vi "Source_File and folder names.vi"() -> (0 "Fixed strings":T1)   [LabVIEW 2020]
uses:
  Typedefs/Fixed strings.ctl
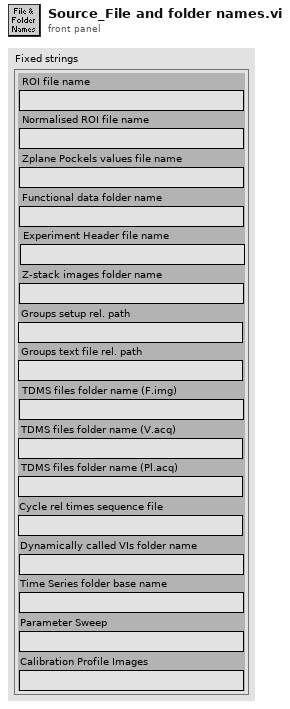
[diagram p1: front panel]
types:
  T1 = typedef "Fixed strings.ctl" = cluster{"ROI file name":string, "Normalised ROI file name":string, "Zplane Pockels values file name":string, "Functional data folder name":string, "Experiment Header file name":string, "Z-stack images folder name":string, "Groups setup rel. path":string, "Groups text file rel. path":string, "TDMS files folder name (F.img)":string, "TDMS files folder name (V.acq)":string, "TDMS files folder name (Pl.acq)":string, "Cycle rel times sequence file":string, "Dynamically called VIs folder name":string, "Time Series folder base name":string, "Parameter Sweep":string, "Calibration Profile Images":string}
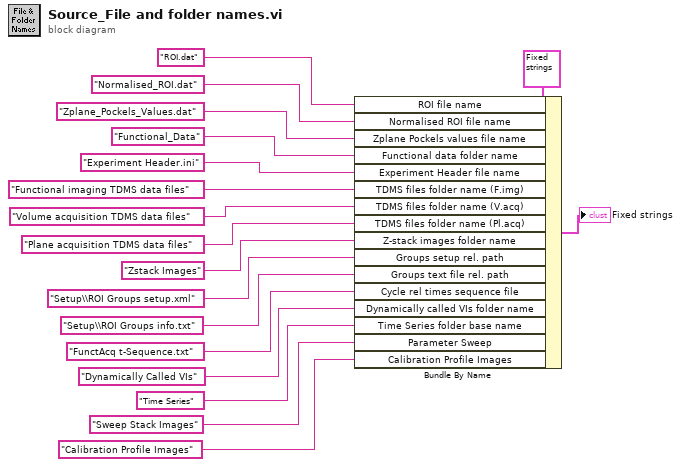
[diagram p0: block diagram]
diagram:
  n1 = Bundle By Name(cluster=T1 {"ROI file name"="", "Normalised ROI file name"="", "Zplane Pockels values file name"="", "Functional data folder name"="", "Experiment Header file name"="", "Z-stack images folder name"="", "Groups setup rel. path"="", "Groups text file rel. path"="", "TDMS files folder name (F.img)"="", "TDMS files folder name (V.acq)"="", "TDMS files folder name (Pl.acq)"="", "Cycle rel times sequence file"="", "Dynamically called VIs folder name"="", "Time Series folder base name"="", "Parameter Sweep"="", "Calibration Profile Images"=""} ("Fixed strings"), "ROI file name"="ROI.dat" ("name or relative path"), "Normalised ROI file name"="Normalised_ROI.dat" ("name or relative path"), "Zplane Pockels values file name"="Zplane_Pockels_Values.dat" ("name or relative path"), "Functional data folder name"="Functional_Data" ("name or relative path"), "Experiment Header file name"="Experiment Header.ini" ("name or relative path"), "TDMS files folder name (F.img)"="Functional imaging TDMS data files" ("name or relative path"), "TDMS files folder name (V.acq)"="Volume acquisition TDMS data files" ("name or relative path"), "TDMS files folder name (Pl.acq)"="Plane acquisition TDMS data files" ("name or relative path"), "Z-stack images folder name"="Zstack Images" ("name or relative path"), "Groups setup rel. path"="Setup\\ROI Groups setup.xml" ("name or relative path"), "Groups text file rel. path"="Setup\\ROI Groups info.txt" ("name or relative path"), "Cycle rel times sequence file"="FunctAcq t-Sequence.txt" ("TDMS files folder name (V.acq)"), "Dynamically called VIs folder name"="Dynamically Called VIs", "Time Series folder base name"="Time Series" ("name or relative path"), "Parameter Sweep"="Sweep Stack Images", "Calibration Profile Images"="Calibration Profile Images" ("Parameter Sweep")) -> (→"Fixed strings":T1)
